vi "LLB Pre-Build CHM Build.vi"(6 "Top Level/Always Included VIs":path[](array[path]), 7 "Main Destination Path":path, 9 "Target Name":string, 10 "Build Specification Name":string, 11 "Project Path":path) -> (0 "error out":errorcluster)   [LabVIEW 2016]
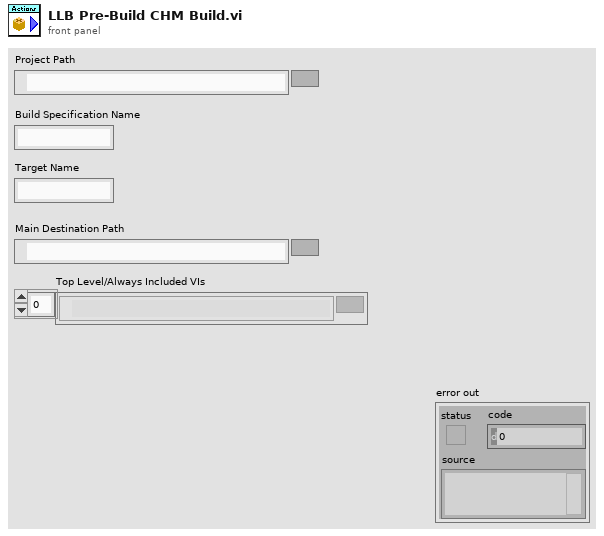
[diagram p1: front panel]
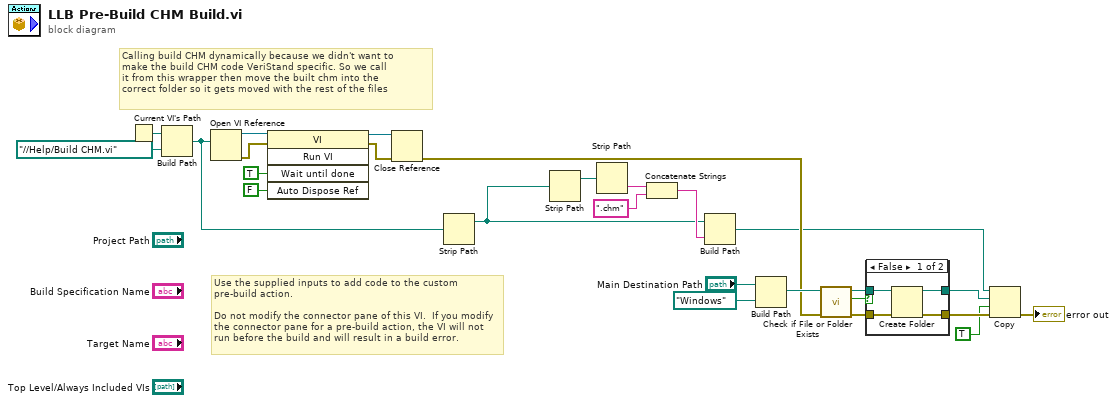
[diagram p0: block diagram]
diagram:
  # "Calling build CHM dynamically because we didn't want to \nmake the build CHM code VeriStand specific. So we call\nit from this wrapper then move the built chm into the\ncorrect folder so it gets moved with the rest of the files"
  # "Use the supplied inputs to add code to the custom pre-build action.\n\nDo not modify the connector pane of this VI.  If you modify the connector pane for a pre-build action, the VI will not run before the build and will result in a build error."
  n1 = Current VI's Path() -> (path=w26:path)
  n2 = Build Path(base path=w26, name or relative path=path "../../Help/Build CHM.vi") -> (appended path=w18:path)
  n3 = Open VI Reference(vi path=w18) -> (vi reference=w24:refnum<vi>, error out=w23:errorcluster)  [unwired: 5 in]
  n4 = invoke class="VI" method="Run VI"(reference=w24, error in=w23, "Wait until done"=TRUE ("Wait Until Done"), "Auto Dispose Ref"=FALSE ("Auto Dispose Reference")) -> (reference out=w20:refnum<vi>, error out=w19:errorcluster)  [unwired: 1 in, 3 out]
  n5 = Close Reference(reference=w20, error in (no error)=w19) -> (error out=w10:errorcluster)
  n6 = Strip Path(path=w18) -> (stripped path=w1:path)  [unwired: 1 out]
  n7 = Strip Path(path=w1) -> (stripped path=w17:path)  [unwired: 1 out]
  n8 = Strip Path(path=w17) -> (name=w16:string)  [unwired: 1 out]
  n9 = Concatenate Strings(w16, ".chm" ("string")) -> (w14:string)
  n10 = Build Path(base path=w1, name or relative path=w14) -> (appended path=w3:path)
  n11 = Build Path(base path="Main Destination Path", name or relative path=path "Windows") -> (appended path=w11:path)
  n12 = call <vilib>:"Check if File or Folder Exists.vi"("error in (no error)"=w10, "path"=w11) -> ("error out"=w7:errorcluster, "file or folder exists?"=w9:bool, "dup path"=w8:path)  [unwired: 7 in]
  n13 = case shown="False" w9 {
    tunnel: w8 -> [w29 w32]
    tunnel: w7 -> [w30 w31]
    tunnel: [w28 w32] -> w5
    tunnel: [w27 w31] -> w6
    frame False {
      n14 = Create Folder(path (use dialog)=w29, error in=w30) -> (created path=w28:path, error out=w27:errorcluster)  [unwired: 1 in, 1 out]
    }
    frame True {
    }
  }
  n15 = Copy(8:w6, 9:TRUE ("overwrite (F)"), 10:w5, 11:w3) -> (0:→"error out":errorcluster)  [unwired: 1 in, 2 out]
